vi "Resonance Detector Process.vi"(8 "error in (no error)":errorcluster, 9 "Best fit guess":dbl[][](array[numeric]) format="%#_4p", 10 "File":path=path "C:/Data/April_2017/042017/ru112_042017.tdms", 11 "Line Detector Configuration":T1={"Peak width guess"=500.0, "Background removal"=enum."High-pass", "Smoothing"=enum."Low-pass", "Smooth window"=200.0, "Relative threshold"=0.2, "Finder algorithm"=enum."Wavelet", "Bgd window"=50000.0, "Spectrum recorder module name"="Spectrum Recorder", "Fit window"=1000.0, "Initial fit guess"=enum."Peak finder", "Follow\npeaks"=FALSE, "Re-sample"=nan} {"Re-sample" format="%#_6pHz"; "Fit window" format="%#_6pHz"; "Bgd window" format="%#_6pHz"; "Smooth window" format="%#_6pHz"; "Peak width guess" format="%#_6pHz"}) -> (0 "error out":errorcluster, 1 "Plots":cluster{"X":dbl[], "Array":dbl[]}[](array[cluster]), 2 "Peaks absolute time":dbl[](array[numeric]), 3 "Best fit results":dbl[][](array[numeric]) format="%#_4p", 4 "Peak Plot":cluster{"Ramp Pattern":dbl[], "X":dbl[]}[](graph), 5 "Peaks":dbl[](array[numeric]) format="%#_4p", 6 "sp time":timestamp, 7 "Good fit?":dbl[](array[numeric]) format="%#_4p")   [LabVIEW 2020]
uses:
  LabActor/Post-Processors/Line Detector/Resonance Detector Configuration.ctl
panel:
  out "File out":path
  # "F0         dF     Ampl   Phase   Xbgrd   Ybgrd    mask"
  # "F0         dF     Ampl   Phase   Xbgrd   Ybgrd"
  # "Peak finder config"
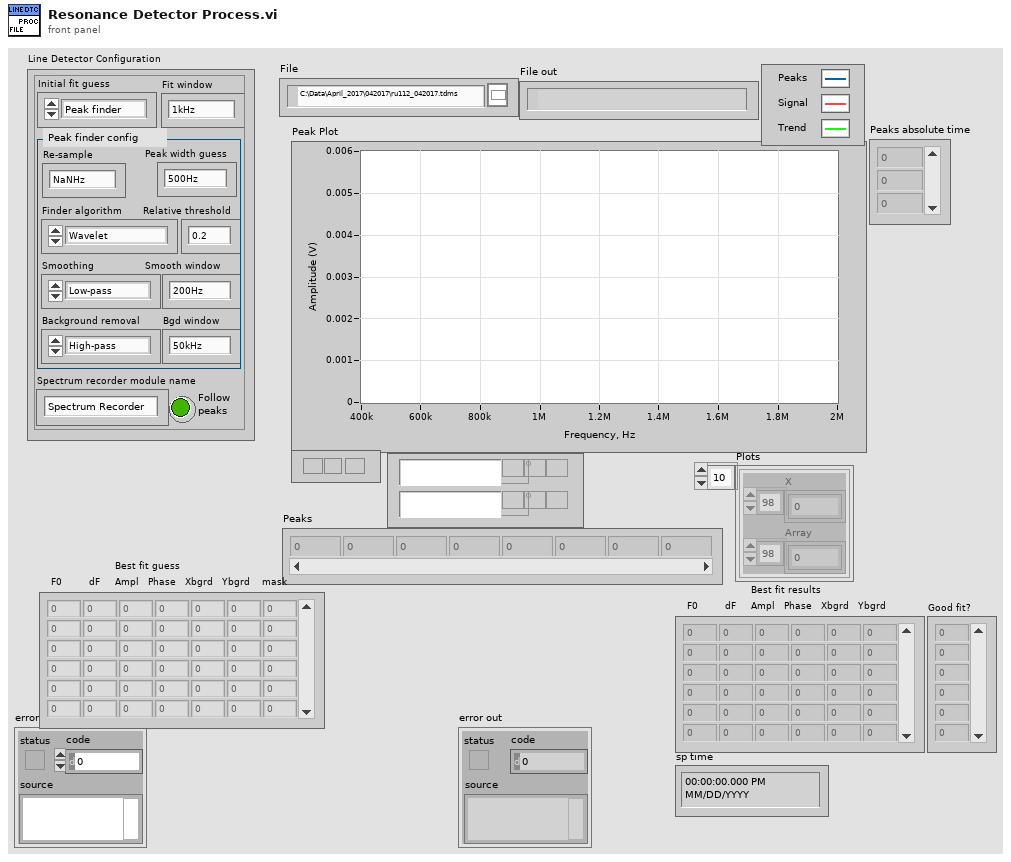
[diagram p1: front panel]
types:
  T1 = typedef "Resonance Detector Configuration.ctl" = cluster{"Peak width guess":dbl, "Background removal":enum16{"NONE", "High-pass", "Detrend"}, "Smoothing":enum16{"NONE", "Low-pass", "Denoise"}, "Smooth window":dbl, "Relative threshold":dbl, "Finder algorithm":enum16{"Basic", "Wavelet", "Wavelet+detrend"}, "Bgd window":dbl, "Spectrum recorder module name":string, "Fit window":dbl, "Initial fit guess":enum16{"Peak finder", "Last fit"}, "Follow\npeaks":bool, "Re-sample":dbl}
  T2 = typedef "Internal Spectrum Configuration.ctl" = cluster{"Start frequency":dbl, "End frequency":dbl, "Coarse step":dbl, "Step duration":dbl, "Red Pitaya address":string, "Open plot \non start":bool, "Fine region centers":dbl[], "Regions width":dbl, "Fine step":dbl, "Pause between scans":dbl, "Clear rgs on start":bool, "Output amplitude":dbl}
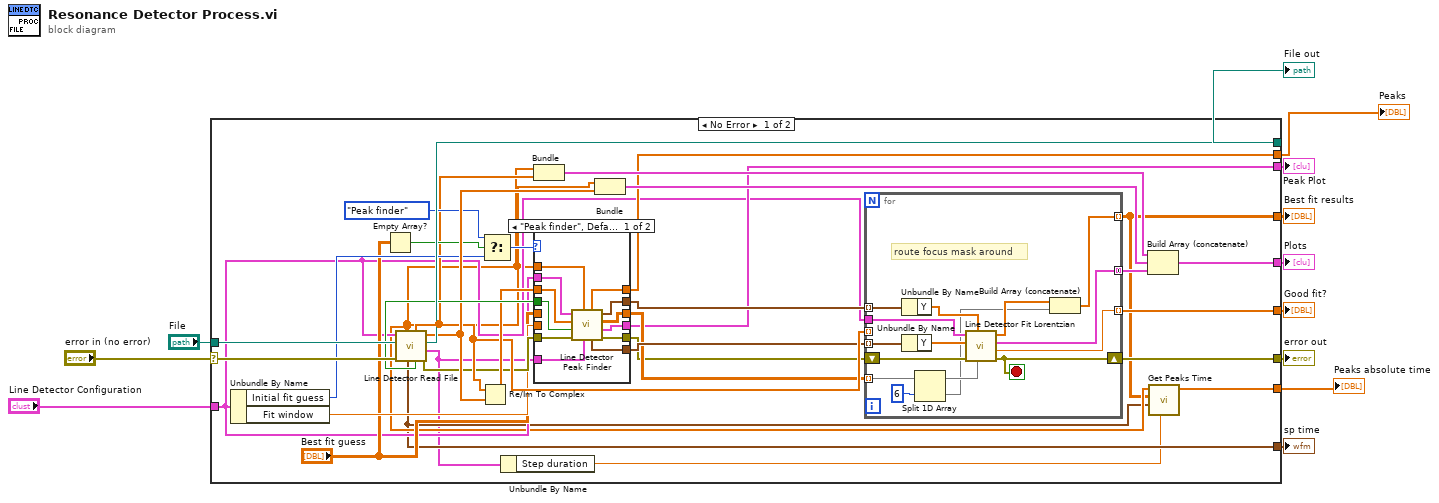
[diagram p0: block diagram]
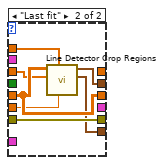
[diagram p2: hidden frame]
diagram:
  n1 = case shown="No Error" "error in (no error)" {
    selector: "error in (no error)" -> [w40 w80]
    tunnel: "File" -> [w41 w81]
    tunnel: [w39 w81] -> w10
    tunnel: "Line Detector Configuration" -> [w19 _]
    tunnel: [w38 w80] -> w8
    tunnel: [w26 _] -> w6
    tunnel: [w16 _] -> w3
    tunnel: [w42 _] -> w7
    tunnel: [w22 _] -> w5
    tunnel: [w17 _] -> w4
    tunnel: [w20 _] -> w2
    tunnel: [w13 _] -> w1
    frame No Error {
      n2 = Unbundle By Name(w19) -> ("Initial fit guess"=w32:enum16{"Peak finder", "Last fit"}, "Fit window"=w23:dbl)
      n3 = Empty Array?(array="Best fit guess") -> (empty?=w34:bool)
      n4 = call "Line Detector Read File.vi"("error in (no error)"=w40, "File"=w41, "Line Detector Configuration"=w19) -> ("error out"=w25:errorcluster, "Internal Spectrum Configuration"=w15:T2, "File out"=w39:path, "Signal Y"=w35:dbl[], "found?"=w37:bool, "Signal X"=w29:dbl[], "sp time"=w17:timestamp, "Frequency"=w18:dbl[])  [unwired: 1 out]
      n5 = Re/Im To Complex(1:w35, 2:w29) -> (0:w36:cdb[])
      n6 = Select(t=enum16{"Peak finder", "Last fit"}."Peak finder" ("Initial fit guess"), s=w34, f=w32) -> (s? t:f=w31:enum16{"Peak finder", "Last fit"})
      n7 = Unbundle By Name(w15) -> ("Step duration"=w14:dbl)
      n8 = Bundle("Frequency"=w18, "Signal X"=w29) -> (w45:cluster{"Frequency":dbl[], "Signal X":dbl[]})  [unwired: 1 in]
      n9 = case shown="\"Peak finder\", Default" w31 {
        tunnel: w19 -> [w57 _]
        tunnel: w18 -> [w56 w63]
        tunnel: w15 -> [w55 _]
        tunnel: w37 -> [w48 _]
        tunnel: w36 -> [w54 w61]
        tunnel: w25 -> [w53 w64]
        tunnel: [w52 w62] -> w27
        tunnel: "Best fit guess" -> [_ w62]
        tunnel: [w51 _] -> w26
        tunnel: [w50 w64] -> w24
        tunnel: [w49 _] -> w22
        tunnel: [w47 w59] -> w30
        tunnel: [w46 w58] -> w28
        tunnel: w23 -> [_ w60]
        frame "Peak finder", Default {
          n10 = call "Line Detector Peak Finder.vi"("Internal Spectrum Configuration"=w55, "Frequency"=w56, "error in (no error)"=w53, "Valid Spectrum Recorder Configuration"=w48, "Signal"=w54, "Line Detector Configuration"=w57) -> ("error out"=w50:errorcluster, "Peak Plot"=w51:cluster{"Ramp Pattern":dbl[], "X":dbl[]}[], "Initial fit guess"=w52:dbl[][], "Regions frequencies"=w47:waveform(dbl)[], "Regions signals"=w46:waveform(cdb)[], "Peaks"=w49:dbl[])
        }
        frame "Last fit" {
          n11 = call "Line Detector Crop Regions.vi"("Region width"=w60, "Frequency"=w63, "Signal"=w61, "Best fit"=w62) -> ("Regions signals"=w58:waveform(cdb)[], "Regions frequencies"=w59:waveform(dbl)[])  [unwired: 6 in]
        }
      }
      n12 = Bundle("Frequency"=w18, "Signal Y"=w35) -> (w44:cluster{"Frequency":dbl[], "Signal Y":dbl[]})  [unwired: 1 in]
      n13 = for {
        tunnel: w19 -> [w79]
        shift-right: [w70] -> w38
        shift-left: w24 -> [w76]
        tunnel: [w67] -> w16 mode=indexing
        tunnel: [w77] -> w43 mode=concatenating
        tunnel: w30 -> [w73] mode=indexing
        tunnel: w29 -> [_] mode=indexing
        tunnel: w28 -> [w75] mode=indexing
        tunnel: w27 -> [w74] mode=indexing
        tunnel: [w65] -> w20 mode=indexing
        stop <- w70 stop-if-true
        # "route focus mask around"
        n14 = Unbundle By Name(w73) -> ("Y"=w72:dbl[])
        n15 = Unbundle By Name(w75) -> ("Y"=w71:cdb[])
        n16 = Split 1D Array(array=w74, index=6) -> (first subarray=w69:dbl[], second subarray=w66:dbl[])
        n17 = call "Line Detector Fit Lorentzian.vi"("Guess"=w69, "Frequency"=w72, "Error In"=w76, "Signal"=w71, "Line Detector Configuration"=w79) -> ("Error Out"=w70:errorcluster, "good fit?"=w65:dbl, "Plot"=w77:cluster{"X":dbl[], "Array":dbl[]}[], "best fit parameters"=w78:dbl[])  [unwired: 3 in]
        n18 = Build Array (concatenate)(w78, w66) -> (w67:dbl[])
      }
      n19 = Build Array (concatenate)(w45, w44, w43) -> (w42:cluster{"X":dbl[], "Array":dbl[]}[])
      n20 = call "Get Peaks Time.vi"("dt"=w14, "sp time"=w17, "Best fit results"=w16, "Frequency"=w18) -> ("Peaks absolute time"=w13:dbl[])  [unwired: 7 in]
    }
    frame Error {
    }
  }
  "error out" <- w8
  "File out" <- w10
  "Plots" <- w7
  "Peak Plot" <- w6
  "Peaks" <- w5
  "sp time" <- w4
  "Best fit results" <- w3
  "Good fit?" <- w2
  "Peaks absolute time" <- w1
